vi "InitBusNumber.vi"(8 "ErrorArray In":errorcluster[](array[cluster]), 10 "clFrontPanelControlRefs In":T1) -> (0 "ErrorArray Out":errorcluster[](array[cluster]), 2 "clFrontPanelControlRefs Out":T1)   [LabVIEW 2014, in "TestFramework.lvlib"]
uses:
  TestFramework.lvlib
  FrontPanel/TypeDefs/clFrontPanelControlRefs.ctl
  FGenPlugins/MyPluginBaseClass/TypeDef/PluginParams.ctl
  WfrmGenerator/WfrmPlugins/EventPluginBaseClass/TypeDefs/dblEvtSignalArray.ctl
  FGenPlugins/MyPluginBaseClass/TypeDef/CreateArbWfrmParams.ctl
  WfrmGenerator/WfrmPlugins/EventPluginBaseClass/TypeDefs/clEvtConfig.ctl
  WfrmGenerator/WfrmModule/PublicAPI/Arguments/Requests/dblEvtParams.ctl
  FGenPlugins/MyPluginBaseClass/TypeDef/ConfigArbWfrmParams.ctl
  FGenPlugins/MyPluginBaseClass/TypeDef/TriggerParams.ctl
  <vilib>/Utility/miscctls.llb/LVStringsAndValuesArrayTypeDef_U8.ctl
  <userlib>/NIST/NISTErrorLib/NISTErrorLib.lvlib
  FGenPlugins/MyPluginBaseClass/NISTFGenPluginsBase.lvclass
  WfrmGenerator/WfrmPlugins/EventPluginBaseClass/BaseWfrmPlugin.lvclass
  WfrmGenerator/WfrmModule/WfrmModule.lvlib
panel:
  # "When you add a control \non the front panel, add a\nreference for it in this\ntype def.  This cluster\nwill hold all of the refer-\nences to the front panel\ncontrols in order to pass\nthese control references \nto subvis."
  # "When you add a control \non the front panel, add a\nreference for it in this\ntype def.  This cluster\nwill hold all of the refer-\nences to the front panel\ncontrols in order to pass\nthese control references \nto subvis."
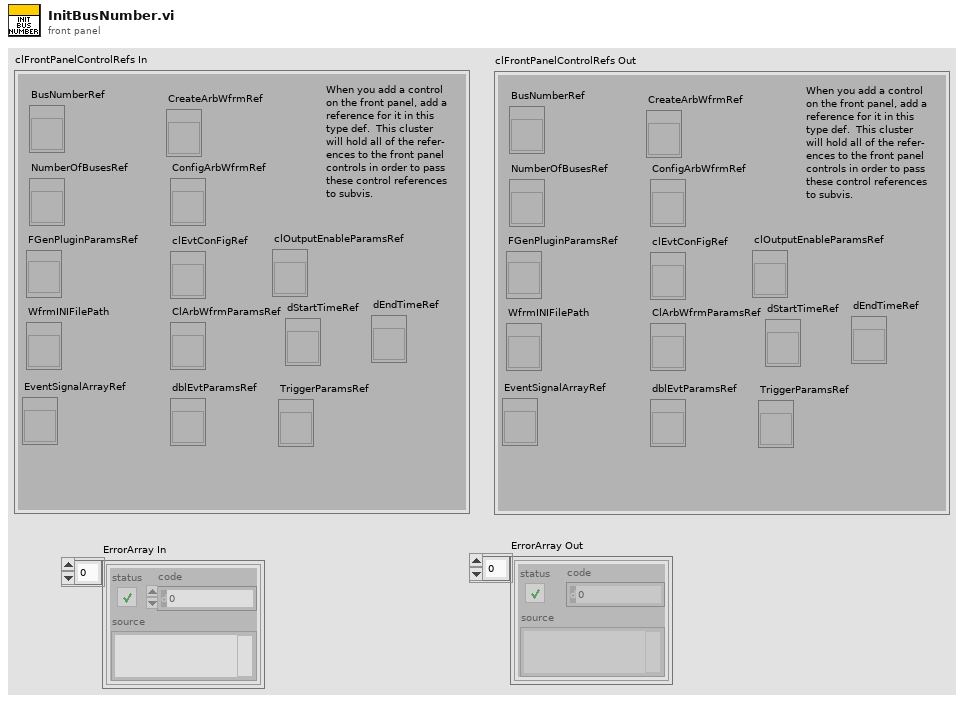
[diagram p1: front panel]
types:
  T1 = typedef "TestFramework.lvlib/clFrontPanelControlRefs.ctl" = cluster{"BusNumberRef":refnum<vi>, "NumberOfBusesRef":refnum<vi>, "FGenPluginParamsRef":refnum<vi>, "WfrmINIFilePath":refnum<vi>, "EventSignalArrayRef":refnum<vi>, "CreateArbWfrmRef":refnum<vi>, "clEvtConFigRef":refnum<vi>, "dblEvtParamsRef":refnum<vi>, "clOutputEnableParamsRef":refnum<vi>, "ConfigArbWfrmRef":refnum<vi>, "ClArbWfrmParamsRef":refnum<vi>, "dStartTimeRef":refnum<vi>, "dEndTimeRef":refnum<vi>, "TriggerParamsRef":refnum<vi>}
  T2 = typedef "LVStringsAndValuesArrayTypeDef_U8.ctl" = cluster{"String":string, "Value":u8}[]
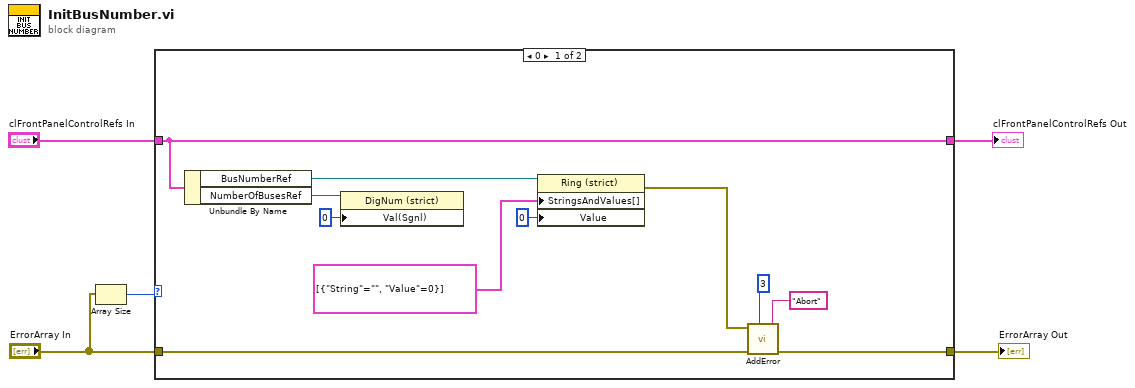
[diagram p0: block diagram]
diagram:
  n1 = Array Size(array="ErrorArray In") -> (size(s)=w5:i32)
  n2 = case shown="0" w5 {
    tunnel: "ErrorArray In" -> [w9 w17]
    tunnel: "clFrontPanelControlRefs In" -> [w16 w18]
    tunnel: [w16 w18] -> w2
    tunnel: [w6 w17] -> w1
    frame 0 {
      n3 = Unbundle By Name(w16) -> ("BusNumberRef"=w13:refnum<vi>, "NumberOfBusesRef"=w15:refnum<vi>)
      n4 = property class="DigNum (strict)"(reference=w15, "Val(Sgnl)"=u8 0 ("Value (Signaling)")) -> ()  [unwired: 1 in, 2 out]
      n5 = property class="Ring (strict)"(reference=w13, "StringsAndValues[]"=T2 [{"String"="", "Value"=0}] ("Strings And Values []"), "Value"=u8 0) -> (error out=w10:errorcluster)  [unwired: 1 in, 1 out]
      n6 = call <userlib>:"AddError.vi"("Severity"="Abort" ("String"), "Priority"=u8 3, "ErrorArray"=w9, "error in (no error)"=w10) -> ("ErrorArray"=w6:errorcluster[])  [unwired: 6 in, 1 out]
    }
    frame 1, Default {
    }
  }
  "clFrontPanelControlRefs Out" <- w2
  "ErrorArray Out" <- w1
